vi "Close.vi"(8 "error in":errorcluster, 11 "CANopen in":refnum<class "CANopen.lvclass">) -> (0 "error out":errorcluster, 3 "CANopen out":refnum<class "CANopen.lvclass">)   [LabVIEW 2024, in "canopen.lvlib" / "CANopen.lvclass"]
uses:
  CANopen.lvclass
  CANopen.lvclass/CANopen.ctl
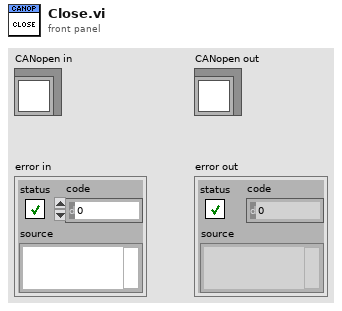
[diagram p1: front panel]
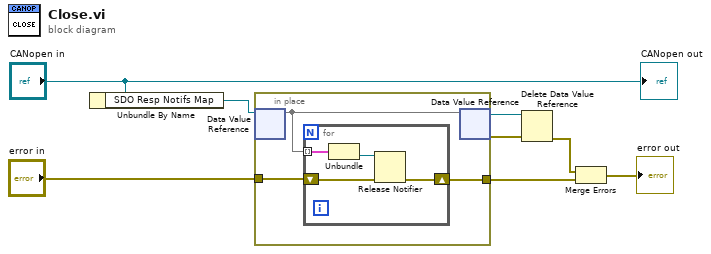
[diagram p0: block diagram]
diagram:
  n1 = Unbundle By Name("CANopen in") -> ("SDO Resp Notifs Map"=w7:refnum<data-value>)
  n2 = in-place {
    in-place-border: [w11] -> w2
    in-place-border: "error in" -> [w10]
    n3 = in-place-dvr #1(w7) -> (w9:map{u32, refnum<notifier>})  [unwired: 1 out]
    n4 = for {
      tunnel: w9 -> [w15] mode=indexing
      shift-right: [w13] -> w11
      shift-left: w10 -> [w12]
      n5 = Unbundle(w15) -> ("notifier out"=w14:refnum<notifier>)  [unwired: 1 out]
      n6 = Release Notifier(notifier=w14, error in (no error)=w12) -> (error out=w13:errorcluster)  [unwired: 1 in, 2 out]
    }
    n7 = in-place-dvr #1(w9) -> (w6:refnum<data-value>, w4:errorcluster)
  }
  n8 = Delete Data Value Reference(data value reference=w6, error in=w4) -> (error out=w3:errorcluster)  [unwired: 1 out]
  n9 = Merge Errors(w3, w2) -> (→"error out":errorcluster)
  "CANopen out" <- "CANopen in"
